vi "S2DS_Welcome.vi"() -> (0 "error out":errorcluster, 1 "Own instrument?":bool, 2 "User info":string[](array[string]))   [LabVIEW 2025]
uses:
  <vilib>/Utility/sysdir.llb/System Directory Type.ctl
panel:
  in  "OK 2":bool
  in  "Logbook path":path
  in  "File index":u32
  in  "File prefix":string
  in  "I have own instruments to use.":bool
  in  "Your email":string
  in  "Session name":string
  in  "Project name*":string(combo)
  in  "Your name*":string(combo)
  out "String":string
  out "substring":string
  in  "OK":bool
  # "Welcome to"
  # "2D SWEEP ..."
  # "* mandatory field"
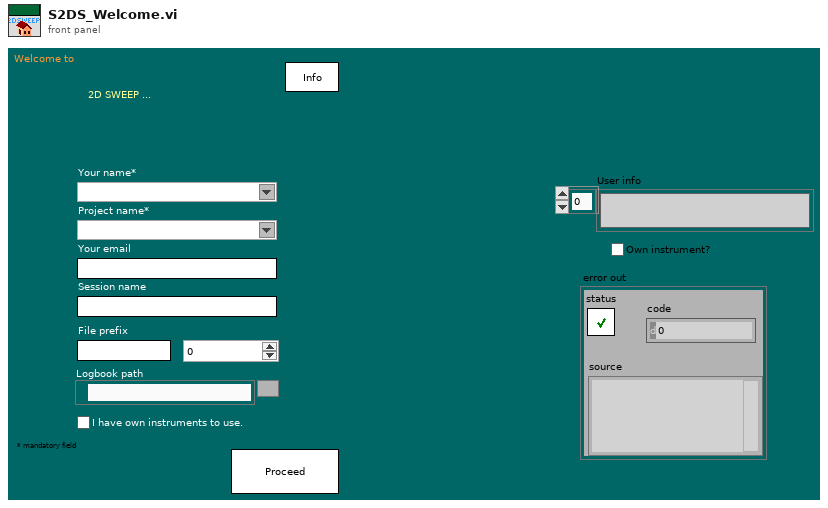
[diagram p1: front panel]
types:
  T1 = typedef "System Directory Type.ctl" = i32
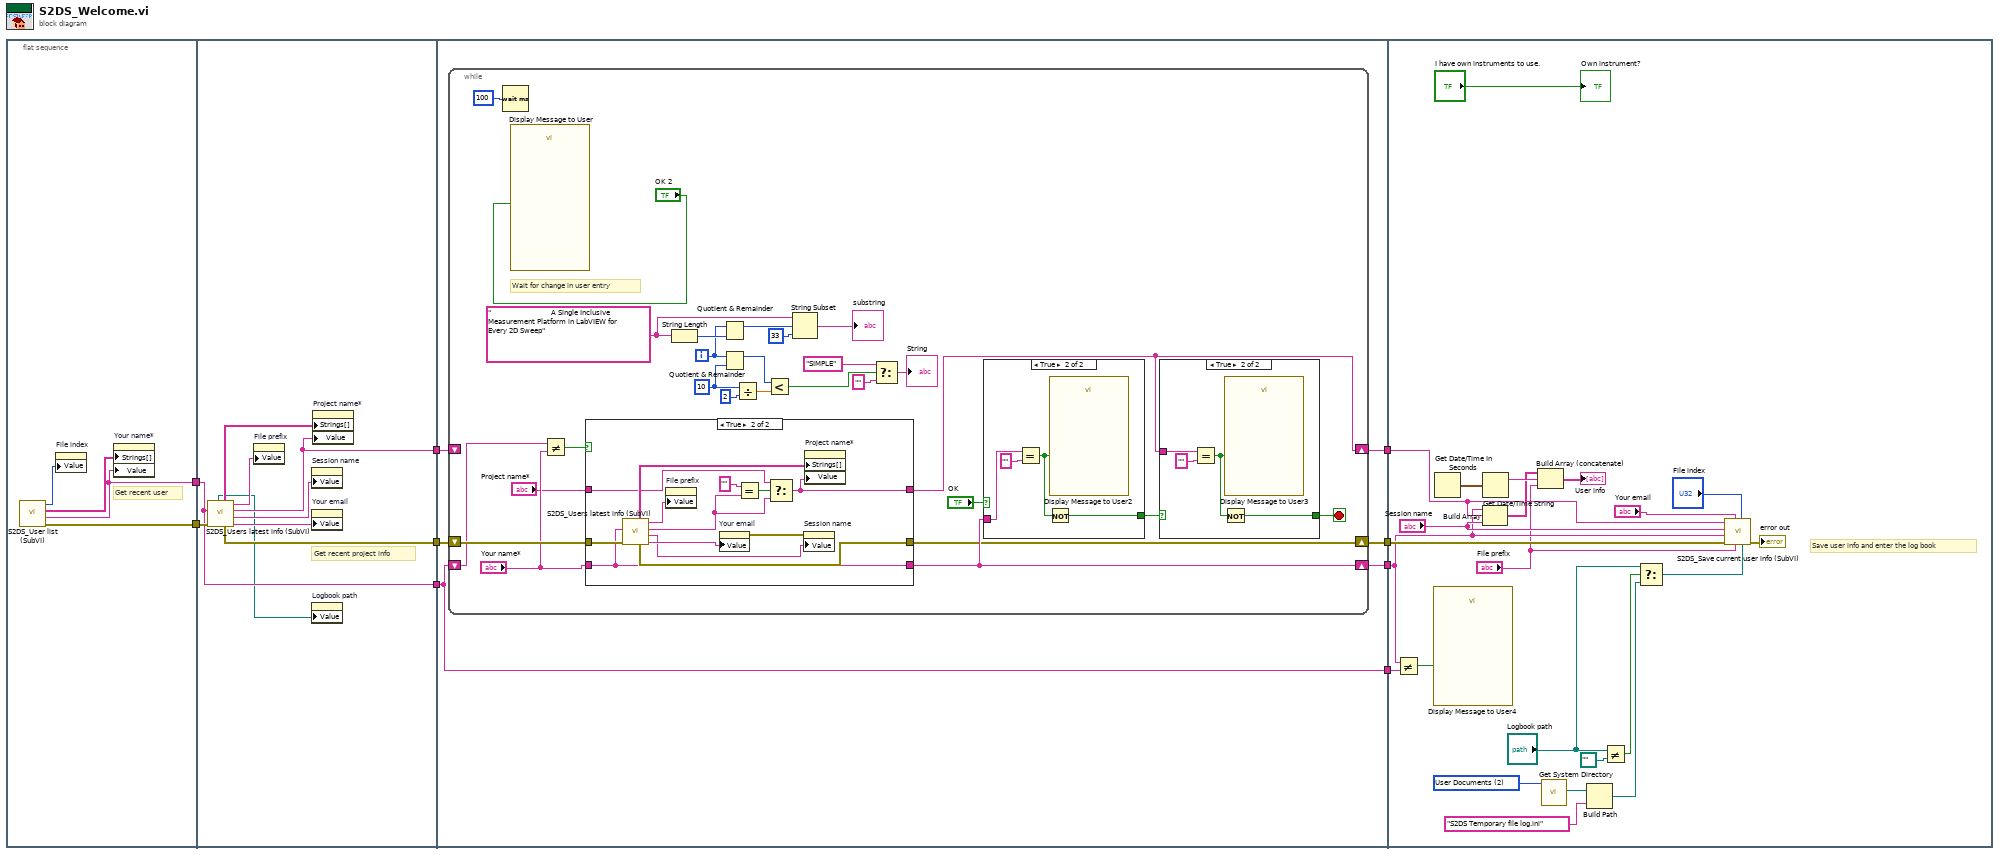
[diagram p0: block diagram]
diagram:
  n1 = flat-sequence {
    tunnel: [w12] -> w7
    tunnel: [w11] -> w6
    tunnel: [w20] -> w9
    tunnel: [w17] -> w8
    tunnel: w7 -> [w18]
    tunnel: w6 -> [w17]
    tunnel: [w16] -> w3
    tunnel: w9 -> [w28]
    tunnel: w8 -> [w23]
    tunnel: [w27] -> w5
    tunnel: [w26] -> w4
    tunnel: w3 -> [w25]
    tunnel: [w24] -> w2
    tunnel: [w23] -> w1
    tunnel: w5 -> [w100]
    tunnel: w4 -> [w94]
    tunnel: w2 -> [w95]
    tunnel: w1 -> [w93]
    frame #0 {
      # "Get recent user"
      n2 = call "S2DS_User list (SubVI).vi"() -> ("error out"=w12:errorcluster, "Current user"=w11:string, "User list"=w13:string[], "File index"=w10:u32)  [unwired: 8 in]
      n3 = property on="File index" class="DigNum (strict)"("Value"=w10) -> ()  [unwired: 2 in, 2 out]
      n4 = property on="Your name*" class="CmbBox"("Strings[]"=w13, "Value"=w11) -> ()  [unwired: 2 in, 2 out]
    }
    frame #1 {
      # "Get recent project info"
      n5 = call "S2DS_Users latest info (SubVI).vi"("error in (no error)"=w18, "User name"=w17) -> ("Email"=w19:string, "Latest session"=w21:string, "Latest project"=w16:string, "File prefix"=w15:string, "error out"=w20:errorcluster, "Project list"=w22:string[], "Logbook path"=w14:path)  [unwired: 3 in]
      n6 = property on="File prefix" class="Str"("Value"=w15) -> ()  [unwired: 2 in, 2 out]
      n7 = property on="Session name" class="Str"("Value"=w21) -> ()  [unwired: 2 in, 2 out]
      n8 = property on="Your email" class="Str"("Value"=w19) -> ()  [unwired: 2 in, 2 out]
      n9 = property on="Logbook path" class="Path"("Value"=w14) -> ()  [unwired: 2 in, 2 out]
      n10 = property on="Project name*" class="CmbBox"("Strings[]"=w22, "Value"=w16) -> ()  [unwired: 2 in, 2 out]
    }
    frame #2 {
      n11 = while {
        shift-right: [w50] -> w26
        shift-left: w23 -> [w54]
        shift-right: [w30] -> w27
        shift-left: w28 -> [w55]
        shift-right: [w48] -> w24
        shift-left: w25 -> [_]
        i -> [w39]
        stop <- w47 stop-if-true
        w37 = 10 ("y")
        w42 = "                              A Single Inclusive Measurement Platform in LabVIEW for Every 2D Sweep" ("string")
        # "Wait for change in user entry"
        n12 = Wait (ms)(milliseconds to wait=u32 100) -> ()  [unwired: 1 out]
        n13 = call "Display Message to User"("Enable"="OK 2") -> ()  [unwired: 9 in, 2 out]
        n14 = Not Equal?(x=w54, y="Your name*") -> (x != y?=w53:bool)
        n15 = case shown="True" w53 {
          tunnel: [w68 w75] -> w50
          tunnel: "Your name*" -> [w68 w75]
          tunnel: w55 -> [w67 w81]
          tunnel: [w67 w80] -> w30
          tunnel: "Project name*" -> [w66 w72]
          tunnel: [w66 w70] -> w48
          frame False {
          }
          frame True {
            n16 = call "S2DS_Users latest info (SubVI).vi"("error in (no error)"=w81, "User name"=w75) -> ("Email"=w78:string, "Latest session"=w76:string, "Latest project"=w71:string, "File prefix"=w69:string, "error out"=w80:errorcluster, "Project list"=w79:string[])  [unwired: 3 in, 1 out]
            n17 = property on="File prefix" class="Str"("Value"=w69) -> ()  [unwired: 2 in, 2 out]
            n18 = property on="Your email" class="Str"("Value"=w78) -> (error out=w77:errorcluster)  [unwired: 2 in, 1 out]
            n19 = Equal?(x="", y=w71) -> (x = y?=w73:bool)
            n20 = Select(t=w72, s=w73, f=w71) -> (s? t:f=w70:string)
            n21 = property on="Session name" class="Str"(error in=w77, "Value"=w76) -> ()  [unwired: 1 in, 2 out]
            n22 = property on="Project name*" class="CmbBox"("Strings[]"=w79, "Value"=w70) -> ()  [unwired: 2 in, 2 out]
          }
        }
        n23 = String Length(string=w42) -> (length=w41:i32)
        n24 = Quotient & Remainder(x=w39, y=w41) -> (x-y*floor(x/y)=w40:i32)  [unwired: 1 out]
        n25 = Quotient & Remainder(x=w39, y=w37) -> (x-y*floor(x/y)=w38:i32)  [unwired: 1 out]
        n26 = Divide(x=w37, y=2) -> (x/y=w35:dbl)
        n27 = Less?(x=w38, y=w35) -> (x < y?=w34:bool)
        n28 = String Subset(string=w42, offset (0)=w40, length (rest)=33 ("length (rest)")) -> (substring=→"substring":string)
        n29 = Select(t="SIMPLE", s=w34, f="") -> (s? t:f=→"String":string)
        n30 = case shown="True" "OK" {
          selector: "OK" -> [w61 _]
          tunnel: w50 -> [_ w65]
          tunnel: [w61 w62] -> w49
          frame False {
          }
          frame True {
            n31 = Equal?(x=w65, y="") -> (x = y?=w63:bool)
            n32 = Not(x=w63) -> (.not. x?=w62:bool)
            n33 = call "Display Message to User2"("Enable"=w63) -> ()  [unwired: 9 in, 2 out]
          }
        }
        n34 = case shown="True" w49 {
          selector: w49 -> [w56 _]
          tunnel: w48 -> [_ w60]
          tunnel: [w56 w57] -> w47
          frame False {
          }
          frame True {
            n35 = Equal?(x=w60, y="") -> (x = y?=w58:bool)
            n36 = Not(x=w58) -> (.not. x?=w57:bool)
            n37 = call "Display Message to User3"("Enable"=w58) -> ()  [unwired: 9 in, 2 out]
          }
        }
      }
    }
    frame #3 {
      w85 = T1 2 items=["User Home"=0, "User Desktop"=1, "User Documents"=2, "User Application Data"=3, "User Preferences"=4, "User Temporary"=5, "Public Documents"=6, "Public Application Data"=7, "Public Preferences"=8, "Public Cache"=13, "System Core Libraries"=9, "System Installed Libraries"=10, "Application Files"=11, "Boot Volume Root"=12] ("system directory type")
      # "Save user info and enter the log book"
      n38 = Not Equal?(x=w94, y=w93) -> (x != y?=w92:bool)
      n39 = call "Display Message to User4"("Enable"=w92) -> ()  [unwired: 9 in, 2 out]
      n40 = Get Date/Time In Seconds() -> (seconds since 1Jan1904=w101:timestamp)
      n41 = Build Array(w94, w95, "Session name") -> (w102:string[])
      n42 = Get Date/Time String(seconds (now)=w101) -> (date string=w103:string)  [unwired: 2 in, 1 out]
      n43 = Build Array (concatenate)(w102, w103, "File prefix") -> (→"User info":string[])
      n44 = call <vilib>:"Get System Directory.vi"("system directory type"=w85) -> ("system directory"=w86:path)  [unwired: 10 in]
      n45 = Build Path(base path=w86, name or relative path="S2DS Temporary file log.ini") -> (appended path=w84:path)
      n46 = Not Equal?(x="Logbook path", y=path "") -> (x != y?=w88:bool)
      n47 = Select(t="Logbook path", s=w88, f=w84) -> (s? t:f=w82:path)
      n48 = call "S2DS_Save current user info (SubVI).vi"("Logbook path"=w82, "File index"="File index", "File prefix"="File prefix", "Your email"="Your email", "error in (no error)"=w100, "Current user"=w94, "Session name"="Session name", "Project name"=w95) -> ("error out"=→"error out":errorcluster)  [unwired: 3 in]
      "Own instrument?" <- "I have own instruments to use."
    }
  }
